vi "createNewInstanceVI.vi"(8 "error in (no error)":errorcluster, 10 "instanceDirectory":path, 11 "PolymorphicInstance in":refnum<class "PolymorphicInstance.lvclass">) -> (0 "error out":errorcluster, 3 "PolymorphicInstance out":refnum<class "PolymorphicInstance.lvclass">)   [LabVIEW 2013, in "PolymorphicInstance.lvclass"]
uses:
  PolymorphicInstance.lvclass
  PolymorphicInstance.lvclass/PolymorphicInstance.ctl
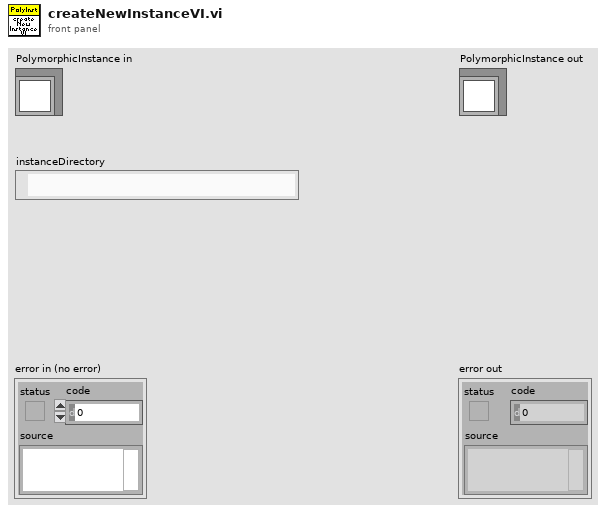
[diagram p1: front panel]
types:
  T1 = enum16{"Invalid Wire Rule", "Required", "Recommended", "Optional", "Dynamic Dispatch"}[]
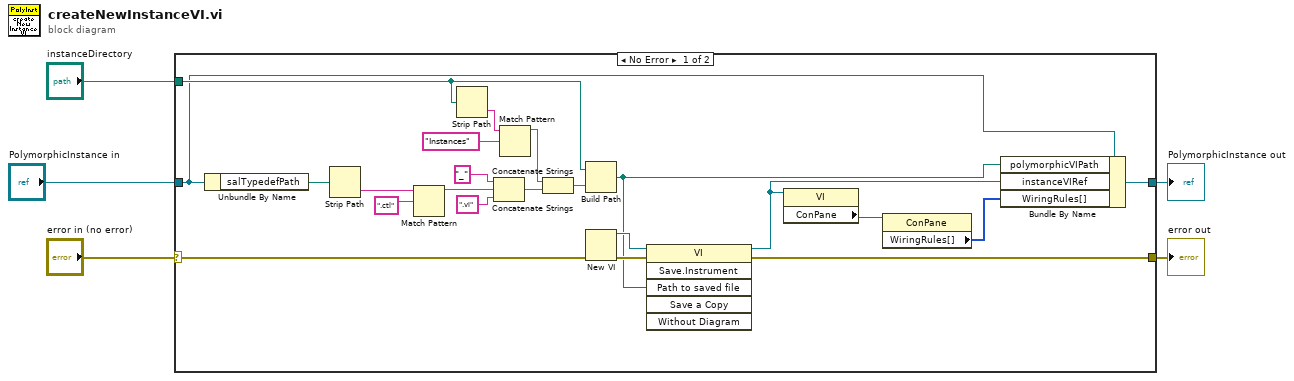
[diagram p0: block diagram]
diagram:
  n1 = case shown="No Error" "error in (no error)" {
    selector: "error in (no error)" -> [w20 w29]
    tunnel: [w19 w29] -> w4
    tunnel: [w18 w28] -> w2
    tunnel: "PolymorphicInstance in" -> [w13 w28]
    tunnel: "instanceDirectory" -> [w21 _]
    frame No Error {
      n2 = Unbundle By Name(w13) -> ("salTypedefPath"=w12:path)
      n3 = Strip Path(path=w12) -> (name=w11:string)  [unwired: 1 out]
      n4 = Match Pattern(string=w11, regular expression=".ctl") -> (before substring=w9:string)  [unwired: 1 in, 3 out]
      n5 = Strip Path(path=w21) -> (name=w27:string)  [unwired: 1 out]
      n6 = Concatenate Strings("_" ("string"), w9, ".vi" ("string")) -> (w7:string)
      n7 = Match Pattern(string=w27, regular expression="Instances") -> (before substring=w25:string)  [unwired: 1 in, 3 out]
      n8 = Concatenate Strings(w25, w7) -> (w24:string)
      n9 = Build Path(base path=w21, name or relative path=w24) -> (appended path=w17:path)
      n10 = New VI(8:w20) -> (0:w22:errorcluster, 3:w23:refnum<vi>)  [unwired: 6 in]
      n11 = invoke class="VI" method="Save.Instrument"(reference=w23, error in=w22, "Path to saved file"=w17) -> (reference out=w16:refnum<vi>, error out=w19:errorcluster)  [unwired: 3 in, 4 out]
      n12 = property class="VI"(reference=w16) -> ("ConPane"=w15:refnum<vi>)  [unwired: 1 in, 2 out]
      n13 = property class="ConPane"(reference=w15) -> ("WiringRules[]"=w14:T1)  [unwired: 1 in, 2 out]
      n14 = Bundle By Name(cluster=w13, "polymorphicVIPath"=w17, "instanceVIRef"=w16, "WiringRules[]"=w14) -> (w18:refnum<class "PolymorphicInstance.lvclass">)
    }
    frame Error {
    }
  }
  "error out" <- w4
  "PolymorphicInstance out" <- w2
